vi "Auto_Routine_BlueStraightThreePieceLeftNoteTRAJ.vi"(8 "error in (no error)":errorcluster) -> (0 "error out":errorcluster)   [LabVIEW 2023]
uses:
  Trajectory/TrajectoryGlobals.vi
  <vilib>/Rock Robotics/WPI/ThirdParty/JAS_Junk/TrajLib/Trajectory_Library.lvlib
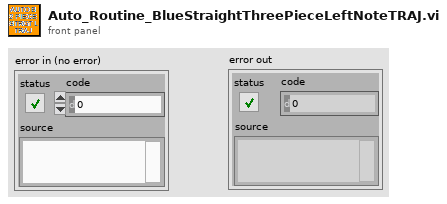
[diagram p1: front panel]
types:
  T1 = typedef "Trajectory_Library.lvlib/TRAJECTORY.ctl" = cluster{"TotalTImeSecs":dbl, "States":T2[]}
  T2 = typedef "Trajectory_Library.lvlib/TRAJ_STATE.ctl" = cluster{"TimeSeconds":dbl, "Velocity":dbl, "Acceleration":dbl, "POSE":T3, "Curvature":dbl}
  T3 = typedef "Trajectory_Library.lvlib/POSE2D.ctl" = cluster{"TRANSLATION":T4, "ROTATION":T5}
  T4 = typedef "Trajectory_Library.lvlib/TRANSLATION2D.ctl" = cluster{"X":dbl, "Y":dbl}
  T5 = typedef "Trajectory_Library.lvlib/ROTATION2D.ctl" = cluster{"VALUE":dbl, "COS":dbl, "SIN":dbl}
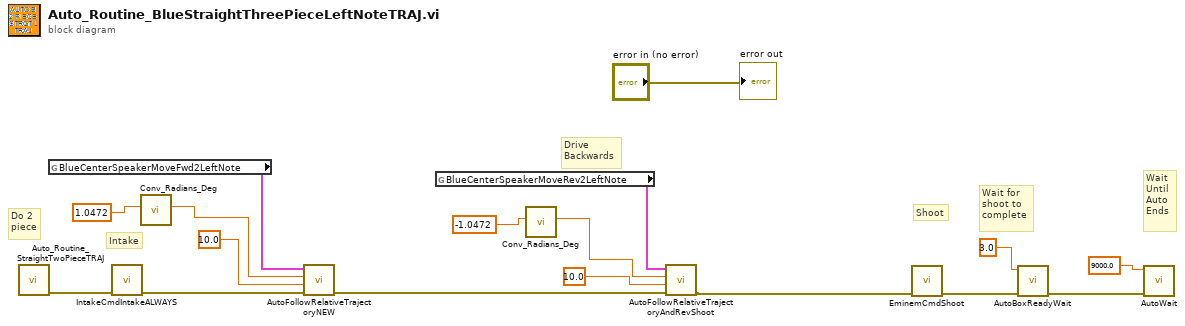
[diagram p0: block diagram]
diagram:
  # "Intake"
  # "Do 2 \npiece"
  # "Wait for\nshoot to\ncomplete"
  # "Shoot"
  # "Drive\nBackwards"
  # "Wait\nUntil\nAuto \nEnds"
  n1 = call "Auto_Routine_StraightTwoPieceTRAJ.vi"() -> ("error out"=w2:errorcluster)  [unwired: 11 in]
  n2 = global read "TrajectoryGlobals.vi" "BlueCenterSpeakerMoveFwd2LeftNote"() -> (w16:T1)
  n3 = call "IntakeCmdIntakeALWAYS.vi"("error in (no error)"=w2) -> ("error out"=w1:errorcluster)  [unwired: 10 in]
  n4 = call <vilib>:"Conv_Radians_Deg.vi"("Radians"=1.0472) -> ("Degrees"=w14:dbl)  [unwired: 10 in]
  n5 = call "AutoFollowRelativeTrajectoryNEW.vi"("error in (no error)"=w1, "TimeOut (s)"=10.0, "End Orientation"=w14, "Trajectory"=w16) -> ("error out"=w4:errorcluster)  [unwired: 7 in]
  n6 = global read "TrajectoryGlobals.vi" "BlueCenterSpeakerMoveRev2LeftNote"() -> (w9:T1)
  n7 = call <vilib>:"Conv_Radians_Deg.vi"("Radians"=-1.0472) -> ("Degrees"=w7:dbl)  [unwired: 10 in]
  n8 = call "AutoFollowRelativeTrajectoryAndRevShoot.vi"("error in (no error)"=w4, "TimeOut (s)"=10.0, "End Orientation"=w7, "Trajectory"=w9) -> ("error out"=w3:errorcluster)  [unwired: 7 in]
  n9 = call "EminemCmdShoot.vi"("error in (no error)"=w3) -> ("error out"=w11:errorcluster)  [unwired: 10 in]
  n10 = call "AutoBoxReadyWait.vi"("error in (no error)"=w11, "TimeOut (s)"=3.0) -> ("error out"=w10:errorcluster)  [unwired: 9 in]
  n11 = call "AutoWait.vi"("error in (no error)"=w10, "TimeOut (s)"=9000.0) -> ()  [unwired: 9 in, 1 out]
  "error out" <- "error in (no error)"
